vi "String to 1D Array 2.vi"(7 "delimiter (,)":string=",", 8 "Error in":errorcluster caption="Error in (no error)", 10 "string":string) -> (0 "Error out":errorcluster, 1 "Array of Strings":string[](array[string])=["sin(x)+2", "VIA(x", "y)", " VIB(z)"])   [LabVIEW 2017, in "API String Arguments Support.lvlib"]
uses:
  API String Arguments Support.lvlib
  <userlib>/_NEVSTOP/Communicable State Machine(CSM)/Communicable State Machine.lvlib
  <userlib>/_NEVSTOP/Communicable State Machine(CSM)/_Shared/CSM Shared.lvlib
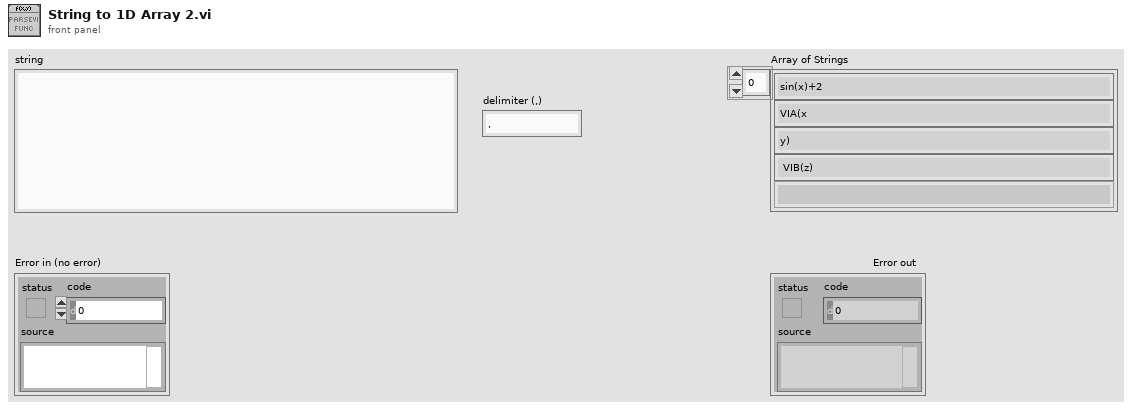
[diagram p1: front panel]
types:
  T1 = enum16{"0x2829 - ()", "0x5B5D - []", "0x7B7D - {}"}
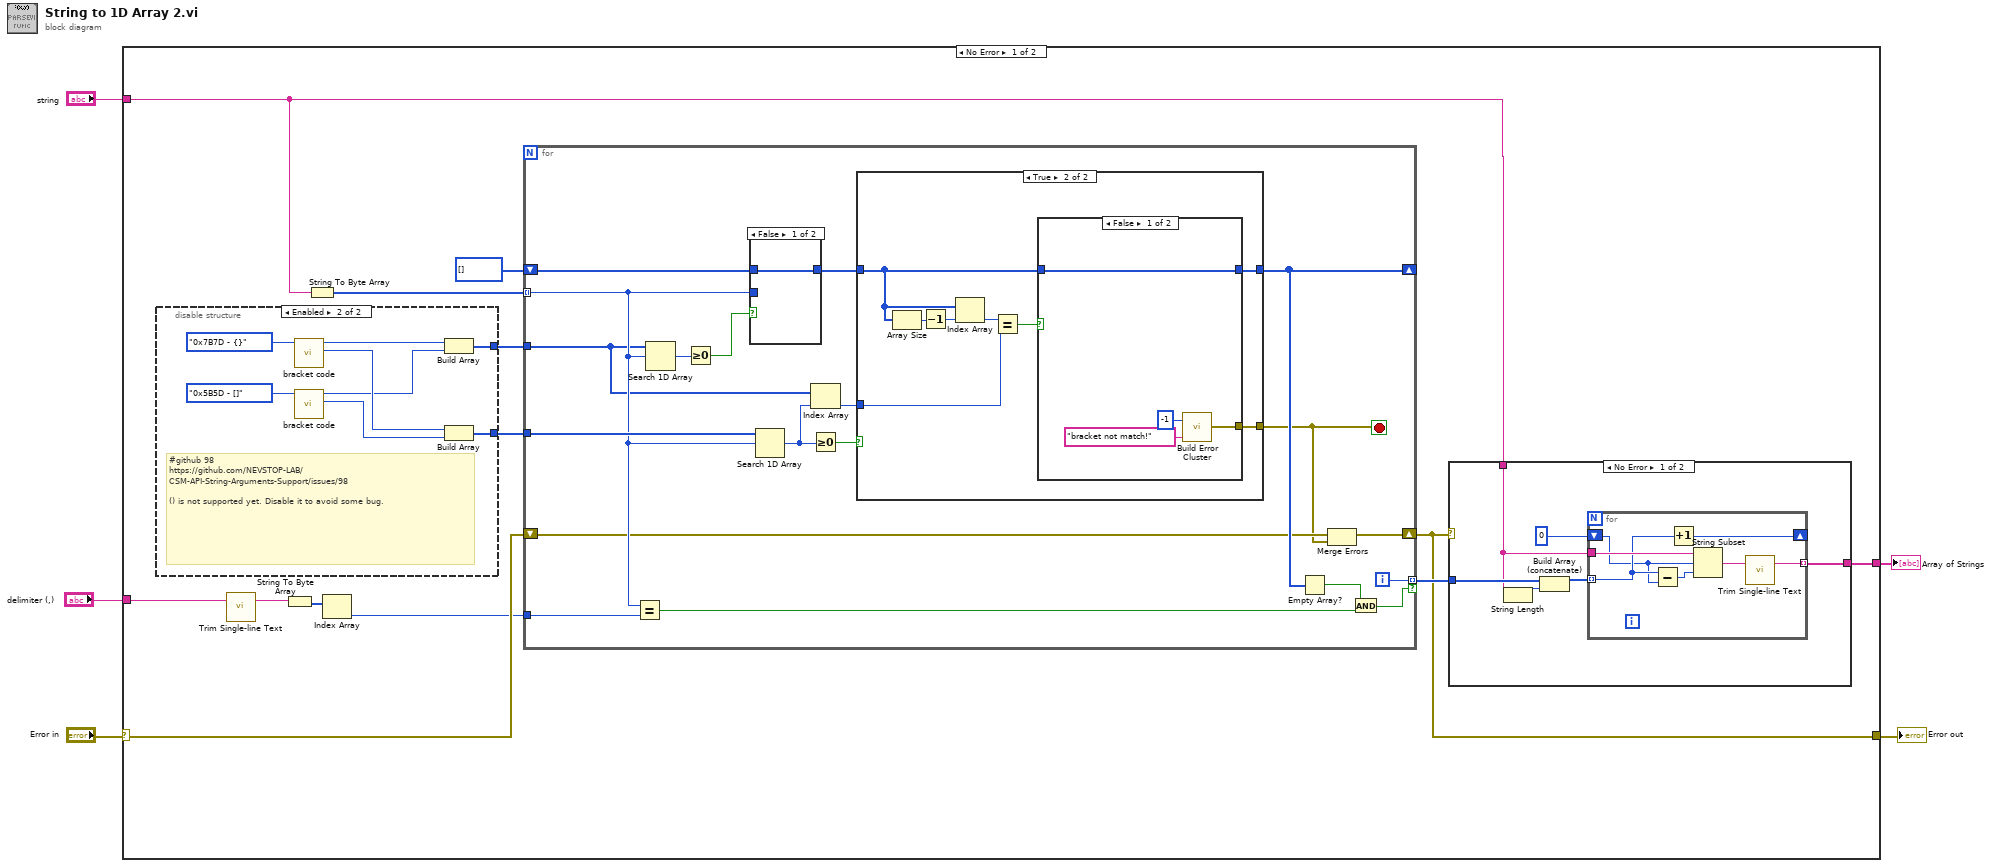
[diagram p0: block diagram]
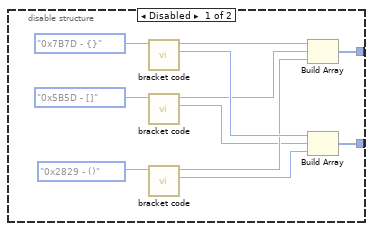
[diagram p2: hidden frame]
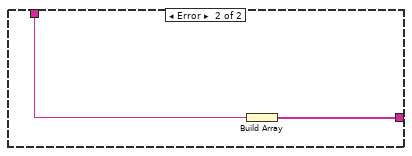
[diagram p3: hidden frame]
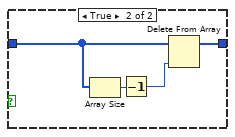
[diagram p5: hidden frame]
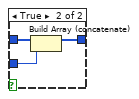
[diagram p6: hidden frame]
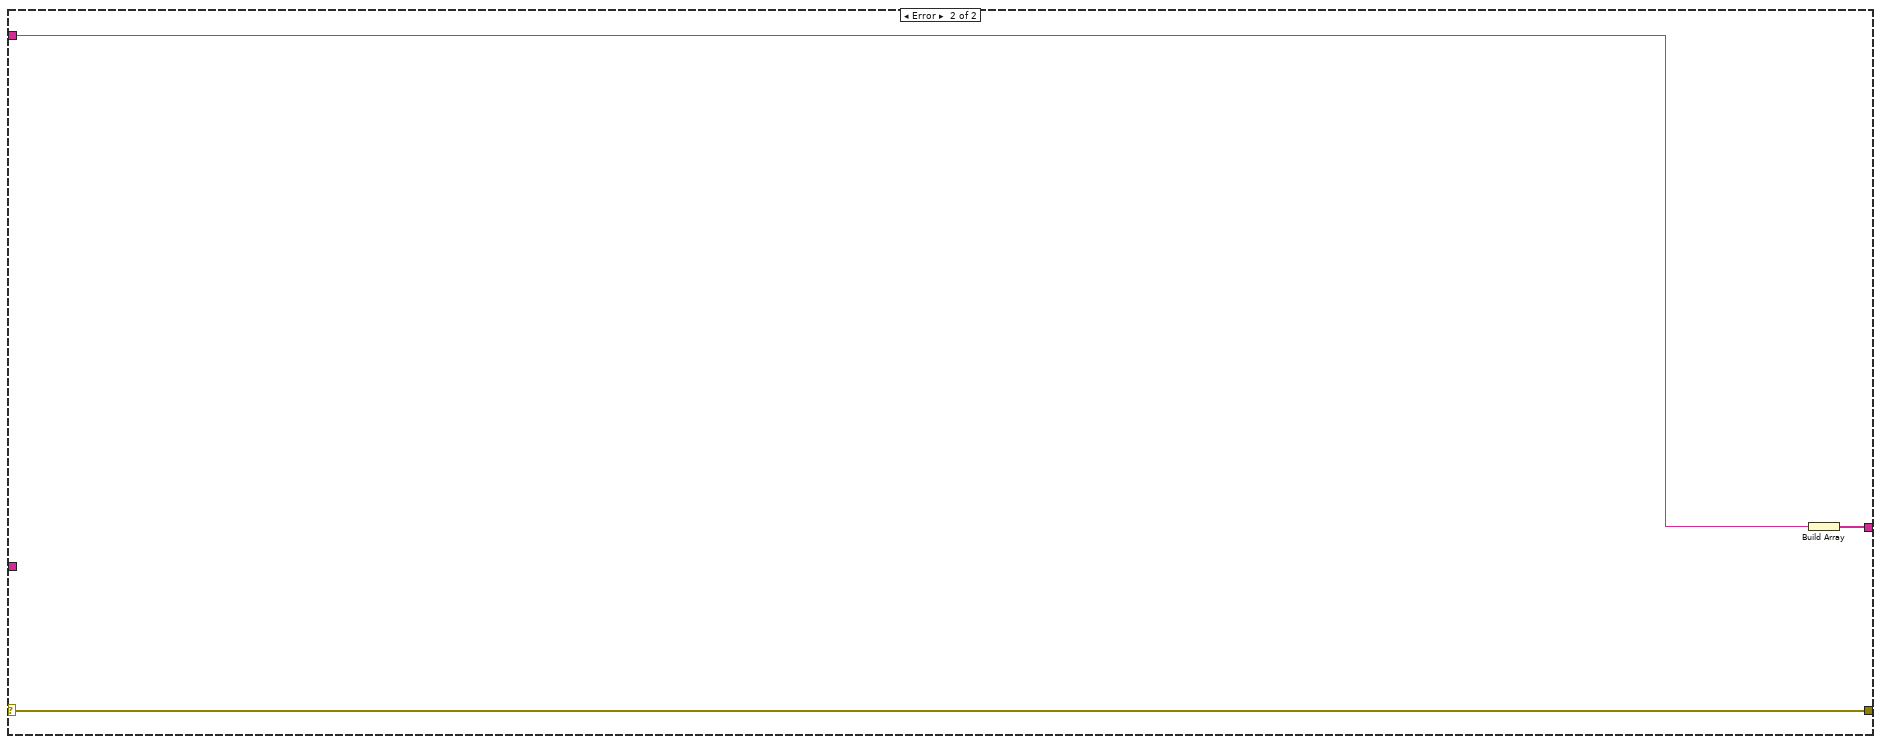
[diagram p7: hidden frame]
diagram:
  n1 = case shown="No Error" "Error in" {
    selector: "Error in" -> [w11 w95]
    tunnel: [w15 w94] -> w5
    tunnel: "string" -> [w14 w93]
    tunnel: [w10 w95] -> w2
    tunnel: "delimiter (,)" -> [w9 _]
    frame No Error {
      n2 = disable-structure shown="Enabled" {
        disable-tunnel: [w25 w34] -> w13
        disable-tunnel: [w19 w30] -> w12
        frame Disabled {
          n3 = call "bracket code.vi"("Enum"=T1."0x7B7D - {}" ("TYPE")) -> ("Numeric"=w24:u8, "Numeric 2"=w28:u8)  [unwired: 9 in]
          n4 = call "bracket code.vi"("Enum"=T1."0x5B5D - []" ("TYPE")) -> ("Numeric"=w21:u8, "Numeric 2"=w23:u8)  [unwired: 9 in]
          n5 = call "bracket code.vi"("Enum"=T1."0x2829 - ()" ("TYPE")) -> ("Numeric"=w20:u8, "Numeric 2"=w22:u8)  [unwired: 9 in]
          n6 = Build Array(w28, w23, w22) -> (w25:u8[])
          n7 = Build Array(w24, w21, w20) -> (w19:u8[])
        }
        frame Enabled {
          # "#github 98\nhttps://github.com/NEVSTOP-LAB/CSM-API-String-Arguments-Support/issues/98\n\n() is not supported yet. Disable it to avoid some bug."
          n8 = call "bracket code.vi"("Enum"=T1."0x7B7D - {}" ("TYPE")) -> ("Numeric"=w33:u8, "Numeric 2"=w36:u8)  [unwired: 9 in]
          n9 = call "bracket code.vi"("Enum"=T1."0x5B5D - []" ("TYPE")) -> ("Numeric"=w31:u8, "Numeric 2"=w32:u8)  [unwired: 9 in]
          n10 = Build Array(w36, w32) -> (w34:u8[])
          n11 = Build Array(w33, w31) -> (w30:u8[])
        }
      }
      n12 = call <userlib>:"Trim Single-line Text.vi"("single-line text"=w9) -> ("trimed text"=w6:string)  [unwired: 2 in]
      n13 = String To Byte Array(string=w6) -> (unsigned byte array=w8:u8[])
      n14 = String To Byte Array(string=w14) -> (unsigned byte array=w17:u8[])
      n15 = Index Array(array=w8) -> (element=w7:u8)  [unwired: 1 in]
      n16 = for {
        tunnel: w17 -> [w59] mode=indexing
        shift-right: [w67] -> _
        shift-left: u8[] [] -> [w70]
        tunnel: [w69] -> w16 mode=indexing if=w66
        tunnel: w13 -> [w54]
        tunnel: w12 -> [w61]
        tunnel: w7 -> [w64]
        shift-right: [w57] -> w10
        shift-left: w11 -> [w58]
        i -> [w69]
        stop <- w56 stop-if-true
        n17 = Equal?(x=w59, y=w64) -> (x = y?=w65:bool)
        n18 = Search 1D Array(1D array=w54, element=w59) -> (index of element=w63:i32)  [unwired: 1 in]
        n19 = Greater Or Equal To 0?(x=w63) -> (x >= 0?=w62:bool)
        n20 = case shown="False" w62 {
          tunnel: w70 -> [w89 w92]
          tunnel: w59 -> [_ w91]
          tunnel: [w89 w90] -> w71
          frame False {
          }
          frame True {
            n21 = Build Array (concatenate)(w92, w91) -> (w90:u8[])
          }
        }
        n22 = Search 1D Array(1D array=w61, element=w59) -> (index of element=w53:i32)  [unwired: 1 in]
        n23 = Index Array(array=w54, index=w53) -> (element=w55:u8)
        n24 = Greater Or Equal To 0?(x=w53) -> (x >= 0?=w60:bool)
        n25 = case shown="True" w60 {
          tunnel: w71 -> [w72 w77]
          tunnel: [w72 w80] -> w67
          tunnel: w55 -> [_ w75]
          tunnel: [_ w73] -> w56
          frame False {
          }
          frame True {
            n26 = Array Size(array=w77) -> (size(s)=w79:i32)
            n27 = Decrement(x=w79) -> (x-1=w78:i32)
            n28 = Index Array(array=w77, index=w78) -> (element=w76:u8)
            n29 = Equal?(x=w76, y=w75) -> (x = y?=w74:bool)
            n30 = case shown="False" w74 {
              tunnel: w77 -> [w84 w87]
              tunnel: [w84 w85] -> w80
              tunnel: [w81 _] -> w73
              frame False {
                n31 = call <userlib>:"Build Error Cluster.vi"("String to Prepend to Source (\"\")"="bracket not match!" ("String to Prepend to source (\"\")"), "Code"=-1 ("code")) -> ("error out"=w81:errorcluster)
              }
              frame True {
                n32 = Array Size(array=w87) -> (size(s)=w88:i32)
                n33 = Decrement(x=w88) -> (x-1=w86:i32)
                n34 = Delete From Array(array=w87, index=w86) -> (array with subset deleted=w85:u8[])  [unwired: 1 in, 1 out]
              }
            }
          }
        }
        n35 = Empty Array?(array=w67) -> (empty?=w68:bool)
        n36 = Merge Errors(w58, w56) -> (w57:errorcluster)
        n37 = And(x=w68, y=w65) -> (x .and. y?=w66:bool)
      }
      n38 = case shown="No Error" w10 {
        tunnel: w16 -> [w43 _]
        tunnel: [w41 w51] -> w15
        tunnel: w14 -> [w38 w52]
        frame No Error {
          n39 = String Length(string=w38) -> (length=w39:i32)
          n40 = Build Array (concatenate)(w43, w39) -> (w40:i32[])
          n41 = for {
            tunnel: w38 -> [w50]
            tunnel: w40 -> [w48] mode=indexing
            tunnel: [w44] -> w41 mode=indexing
            shift-right: [w45] -> _
            shift-left: 0 ("Numeric") -> [w46]
            n42 = Subtract(x=w48, y=w46) -> (x-y=w47:i32)
            n43 = Increment(x=w48) -> (x+1=w45:i32)
            n44 = String Subset(string=w50, offset (0)=w46, length (rest)=w47) -> (substring=w49:string)
            n45 = call <userlib>:"Trim Single-line Text.vi"("single-line text"=w49) -> ("trimed text"=w44:string)  [unwired: 2 in]
          }
        }
        frame Error {
          n46 = Build Array(w52) -> (w51:string[])
        }
      }
    }
    frame Error {
      n47 = Build Array(w93) -> (w94:string[])
    }
  }
  "Array of Strings" <- w5
  "Error out" <- w2
